vi "FPGA Main.vi"() -> ()   [LabVIEW 2021]
uses:
  <vilib>/rvi/Emulation/niFpgaGetClockAttributes.vi
  <vilib>/rvi/Emulation/niFpgaSctlEmulationGetInTimedLoop.vi
  <vilib>/rvi/Emulation/niFpgaEmulationReportErrorSimple.vi
  <vilib>/rvi/eio/common/nirviEmuTemplateMethod_errors.vi
  <vilib>/rvi/Emulation/niFpgaCriticalErrorInLSC.vi
  <vilib>/eio/EIONode/EIONode.xnode
panel:
  in  "Led0":bool
  out "Button0":bool
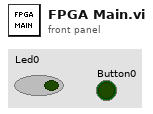
[diagram p1: front panel]
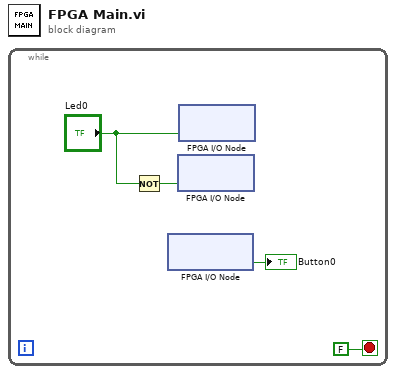
[diagram p0: block diagram]
diagram:
  n1 = while {
    stop <- FALSE stop-if-true
    n2 = Not(x="Led0") -> (.not. x?=w2:bool)
    n3 = xnode "FPGA I/O Node"() -> ("Button0"=→"Button0":bool)  [unwired: 1 in, 1 out]
    n4 = xnode "FPGA I/O Node"("LED3"=w2) -> ()  [unwired: 1 in, 1 out]
    n5 = xnode "FPGA I/O Node"("LED0"="Led0") -> ()  [unwired: 1 in, 1 out]
  }
